vi "ProcessMatlabEvents.vi"(8 "Event Wait timeout":i32=10, 11 "ExperimentID":string) -> ()   [LabVIEW 2017]
uses:
  Types/MethodInvokeInfo.ctl
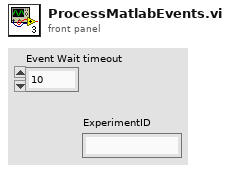
[diagram p1: front panel]
types:
  T1 = typedef "MethodInvokeInfo.ctl" = cluster{"Method Name":string, "Arguments":variant}
  T2 = typedef "MatlabDataBundle.ctl" = cluster{"MatlabType":T3, "Value":variant, "Name":string}
  T3 = typedef "MatlabDataType.ctl" = enum16{"NotAMatlabType", "Real", "Complex", "String", "Boolean"}
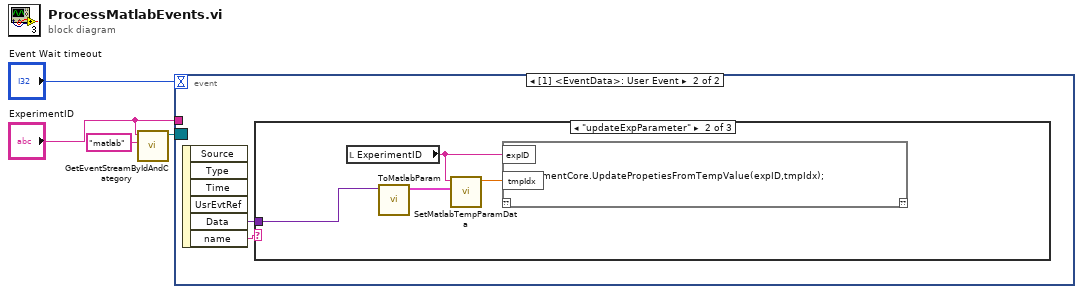
[diagram p0: block diagram]
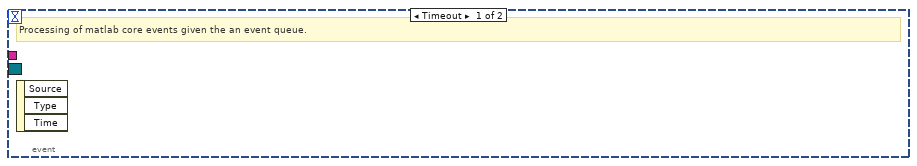
[diagram p2: hidden frame]
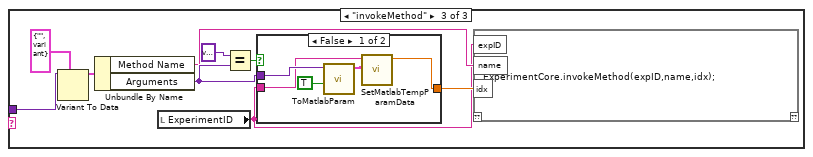
[diagram p4: hidden frame]
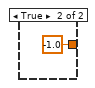
[diagram p5: hidden frame]
diagram:
  n1 = call "GetEventStreamByIdAndCategory.vi"("Category"="matlab", "ID"="ExperimentID") -> ("Event Registration Refnum out"=w4:refnum<event-registration>)  [unwired: 8 in, 1 out]
  n2 = event shown="[1] <EventData>: User Event" {
    selector: w4 -> [_ _]
    dyn-events: _ -> [_ _]
    timeout: "Event Wait timeout" -> [_ _]
    tunnel: "ExperimentID" -> [_ _]
    event Timeout {
      # "Processing of matlab core events given the an event queue."
      n3 = event-data() -> ()  [unwired: 1 in, 3 out]
    }
    event User Event {
      n4 = event-data() -> ("Data"=w5:variant, "name"=w6:string)  [unwired: 1 in, 4 out]
      n5 = case shown="\"updateExpParameter\"" w6 {
        tunnel: w5 -> [_ w10 w18]
        frame "False", Default {
        }
        frame "updateExpParameter" {
          n6 = local read "ExperimentID"() -> (w8:string)
          n7 = call "ToMatlabParam.vi"("Value"=w10) -> ("Matlab Param Data"=w9:T2[])  [unwired: 10 in]
          n8 = call "SetMatlabTempParamData.vi"("Matlab param data"=w9, "ExperimentID"=w8) -> ("index out"=w7:dbl)  [unwired: 9 in]
          n9 = script code="ExperimentCore.UpdatePropetiesFromTempValue(expID,tmpIdx);"("expID"=w8, "tmpIdx"=w7) -> ()  [unwired: 1 in, 1 out]
        }
        frame "invokeMethod" {
          n10 = Variant To Data(type=T1 {"Method Name"="", "Arguments"=variant} ("Method Invoke Info"), Variant=w18) -> (data=w17:T1)  [unwired: 1 in, 1 out]
          n11 = Unbundle By Name(w17) -> ("Method Name"=w12:string, "Arguments"=w13:variant)
          n12 = local read "ExperimentID"() -> (w11:string)
          n13 = Equal?(x=variant, y=w13) -> (x = y?=w14:bool)
          n14 = case shown="False" w14 {
            tunnel: [w22 -1.0] -> w15
            tunnel: w13 -> [w23 _]
            tunnel: w11 -> [w20 _]
            frame False {
              n15 = call "ToMatlabParam.vi"("IgnoreContainerName"=TRUE, "Value"=w23) -> ("Matlab Param Data"=w24:T2[])  [unwired: 9 in]
              n16 = call "SetMatlabTempParamData.vi"("Matlab param data"=w24, "ExperimentID"=w20) -> ("index out"=w22:dbl)  [unwired: 9 in]
            }
            frame True {
            }
          }
          n17 = script code="ExperimentCore.invokeMethod(expID,name,idx);"("expID"=w11, "name"=w12, "idx"=w15) -> ()  [unwired: 1 in, 1 out]
        }
      }
    }
  }
